vi "Dashboard Main.vi"() -> ()   [LabVIEW 2015]
uses:
  PositionSelect.ctl
  DefenseSelect.ctl
  <vilib>/Utility/miscctls.llb/LVRowAndColumnTypeDef.ctl
  <vilib>/event_ctls.llb/eventvkey.ctl
  <vilib>/Rock Robotics/WPI/Dashboard/WPI_DashboardLogging Global.vi
  <vilib>/Rock Robotics/Network Tables/NT Read Numeric Array.vi
  <vilib>/Rock Robotics/Network Tables/NT Read Boolean.vi
  <vilib>/Rock Robotics/Network Tables/NT Write Numeric Array.vi
  <vilib>/Utility/config.llb/Write Key (String).vi
  <vilib>/Utility/config.llb/Write Key (I32).vi
  <vilib>/Utility/config.llb/NI_LVConfig.lvlib
panel:
  in  "TCP":refnum<k5>
  in  "Rec Mode":enum32{"Stop", "Record", "Playback"}(radio)
  in  "Vision":u16(ring) items=["Camera Off", "USB Camera SW", "USB Camera HW", "IP Camera"]
  out "Camera IP":string
  out "Image Message":string="Timeout in Camera Communications"
  in  "Dashboard Tab":T1(tab)
  in  "Select Auto":string(combo)
  out "NT Connection":bool
  in  "Camera Settings":T2={"Frame Rate"=30, "Compression"=30, "Size"=1} {"Frame Rate" scale=1.0..30.0; "Size" items=["640x480", "320x240", "160x120"]}
  out "MotorChart R":cluster{"Numeric":dbl, "Numeric":dbl}(graph)
  out "MotorChart L":T3(graph)
  out "MotorSliders R":cluster{"MotorSlide1":dbl, "MotorSlide2":dbl} {"MotorSlide2" scale=-1.0..1.0 scale format="%#_2e"; "MotorSlide1" scale=-1.0..1.0 scale format="%#_2e"}
  out "MotorSliders L":T4 {"MotorSlide4 2" scale=0.0..14.0 scale format="%#_2e"; "MotorSlide2" scale=-1.0..1.0 scale format="%#_2e"; "MotorSlide1" scale=-1.0..1.0 scale format="%#_2e"}
  out "JS1 Z":dbl(slide) scale=-1.0..1.0 scale format="%#_2e"
  out "JS1 Graph":cluster{"X":dbl, "Y":dbl}[](graph)
  out "JS1 Buttons":T5
  out "JS2 Z":dbl(slide) scale=-1.0..1.0 scale format="%#_2e"
  out "JS2 Graph":cluster{"X":dbl, "Y":dbl}[](graph)
  out "JS2 Buttons":T5
  out "Mode":T6(ring)=enum."Auto Disabled"
  in  "DB Camera Config":bool
  out "fps":dbl format="%#.1g"
  out "Mbps":dbl format="%#.1g"
  out "Mbps LED":bool
  in  "DB/String 9":string
  in  "DB/String 8":string
  in  "DB/String 7":string
  in  "DB/String 6":string
  in  "DB/String 5":string
  in  "DB/String 4":string
  in  "DB/String 3":string
  in  "DB/String 2":string
  in  "DB/String 1":string
  in  "DB/String 0":string
  in  "DB/Slider 0":dbl(slide) scale=0.0..5.0
  in  "DB/Slider 1":dbl(slide) scale=0.0..5.0
  in  "DB/Slider 2":dbl(slide) scale=0.0..5.0
  in  "DB/Slider 3":dbl(slide) scale=0.0..5.0
  out "DB/LED 3":bool
  out "DB/LED 2":bool
  out "DB/LED 1":bool
  out "DB/LED 0":bool
  in  "DB/Button 3":bool
  in  "DB/Button 2":bool
  in  "DB/Button 1":bool
  in  "DB/Button 0":bool caption="New Name"
  in  "Defense Select":T7
  out "RightEncoder":dbl
  out "LeftEncoder":dbl
  in  "Position Select":T8=enum."1 (Wall)"
  out "Yaw":dbl
  out "Case":dbl
  out "EXIT":bool
  out "CameraSwivel":dbl
  out "CameraTilt":dbl
  out "Defense Select Out":T7
  out "Position Select Out":T8=enum."1 (Wall)"
  out "Roll":dbl
  out "Pitch":dbl
  out "Photoeye\nBeam Broken?":bool
  out "Climb Encoder":dbl
  in  "Test Slider":dbl(slide) scale=0.0..100.0 scale format="%#_3g"
  in  "On/Off":bool caption="Solenoid"
  in  "Test Name":u16(ring) items=["Select the test to run..."]
  in  "Test Tree":string(tree)
  in  "Motor":cluster{"Value":dbl, "Enable":bool} {"Value" scale=-1.0..1.0 scale format="%#_3g"}
  out "Progress":T9 {"Test Progress" scale=0.0..100.0}
  in  "Rev/Fwd":cluster{"Forward":bool, "Reverse":bool}
  in  "Test Ring":u16(ring) items=["Monochrome", "Color"]
  out "Cmd Status":string
  in  "Execute Command":bool
  in  "Command Params":string[][](table)
  in  "Command Selection":i32(listbox)
  in  "CheckList":i32(listbox)
  out "Tree":string(tree)
  out "Camera Image":T10(plugin-control)
  out "Background":bool
  # "Left"
  # "Front"
  # "Right"
  # "Battery"
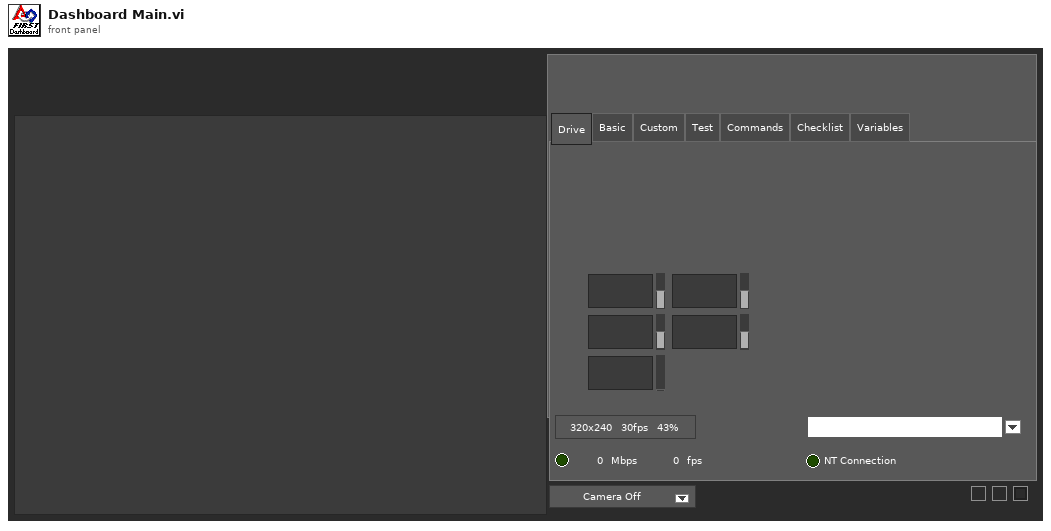
[diagram p1: front panel]
types:
  T1 = enum32{"Drive", "Basic", "Custom", "Test", "Commands", "Checklist", "Variables"}
  T2 = cluster{"Frame Rate":i32, "Compression":i32, "Size":u16}
  T3 = cluster{"Numeric":dbl, "Numeric":dbl, "Battery V":dbl}
  T4 = cluster{"MotorSlide1":dbl, "MotorSlide2":dbl, "MotorSlide4 2":dbl}
  T5 = cluster{bool, bool, bool, bool, bool, bool, bool, bool, bool, bool, bool, bool}
  T6 = enum8{"Tele-Op Disabled", "Tele-Op Enabled", "Auto Disabled", "Auto Enabled", "Test Disabled", "Test Enabled", "Disconnected", "No Code", "E-Stop"}
  T7 = typedef "DefenseSelect.ctl" = enum16{"Low Bar", "Moat", "Rough Terrain", "Rock Wall", "Ramparts", "Portcullis", "Cheval de Frise"}
  T8 = typedef "PositionSelect.ctl" = enum16{"Don't Move", "1 (Wall)", "2", "3", "4", "5", "CrossOnly"}
  T9 = cluster{"Test Progress":u8, "Test Progress Text":string}
  T10 = typedef "IMAQ Image.ctl" = refnum<image>
  T11 = cluster{"IDs":cluster{"RPC field ID":u16, "Unique ID":u16}, "String":string}
  T12 = enum32{"Drive", "Basic", "Custom", "Test", "Checklist", "Variables"}
  T13 = typedef "Image Type" = u32
  T14 = cluster{"Camera Image":refnum<vi>, "Dashboard Tab":refnum<vi>, "Background":refnum<vi>, "Vision":refnum<vi>, "Rec Mode":refnum<vi>, "Test Slider":refnum<vi>, "On/Off ":refnum<vi>, "Test Ring":refnum<vi>, "Rev/Fwd":refnum<vi>, "Test Name":refnum<vi>, "Motor":refnum<vi>, "Progress":refnum<vi>, "CheckList":refnum<vi>, "Tree":refnum<vi>, "Test Tree":refnum<vi>, "Command Params":refnum<vi>, "Command Selection":refnum<vi>, "Execute Command":refnum<vi>, "Cmd Status":refnum<vi>}
  T15 = cluster{"Error Strings":string, "Disable Counts":cluster{u16, u16}, "Rail Faults":cluster{u16, u16, u16}, "Robot IP":string, "DB Mode":u8, "Event Info":cluster{"Name":string, "Type":u8, "Number":u16, "Replay":u8}, "Camera Addr":string}
  T16 = cluster{"Storage":cluster{"Disk Free":u64, "RAM Block":u32, "RAM free":u32}, "CPU Utilization":cluster{"CPU % ISR":sgl, "CPU % Time Crit":sgl, "CPU % Timed Str":sgl, "CPU % High":sgl, "CPU % Above":sgl, "CPU % Normal":sgl, "CPU % Low":sgl}, "CAN":cluster{"% Bus Utilization":sgl, "Bus Off Cnt":u32, "TX_FIFO Full Cnt":u32, "Receive Error Cnt":u8, "Transmit Error Cnt":u8}, "HID":cluster{"HID Outputs":u32, "Rumble Low":u16, "Rumble High":u16}[]}
  T17 = cluster{"Status bits":cluster{"Test Mode":bool, "Autonomous":bool, "Enabled":bool, "Code Start":bool, "Brownout":bool, "Reserved 2":bool, "Reserved 3":bool, "E-Stop":bool}, "Code Trace":cluster{"Disabled":bool, "TeleOp":bool, "Auto":bool, "Test":bool}, "Controller Type":enum16{"unknown", "cRIO", "roboRio"}, "Code?":enum16{"unknown", "noCode", "code"}, "Battery V":dbl}
  T18 = cluster{"Control Bits":cluster{"TestMode":bool, "Autonomous":bool, "Enabled":bool, "FMS Present":bool, bool, bool, bool, "E-Stop":bool}, "Team Station ":u8, "Countdown":sgl, "Joystick Values":cluster{"Axes":dbl[], "Buttons":bool[], "POVs":i16[]}[]}
  T19 = cluster{"Axes":dbl[], "Buttons":bool[], "POVs":i16[]}[]
  T20 = cluster{"Axes":dbl[], "Buttons":bool[], "POVs":i16[]}
  T21 = cluster{"Buttons[0]":bool, "Buttons[1]":bool, "Buttons[2]":bool, "Buttons[3]":bool, "Buttons[4]":bool, "Buttons[5]":bool, "Buttons[6]":bool, "Buttons[7]":bool, "Buttons[8]":bool, "Buttons[9]":bool, "Buttons[10]":bool, "Buttons[11]":bool}
  T22 = typedef "NI_LVConfig.lvlib/Config Data RefNum.ctl" = refnum<k1>
  T23 = cluster{"Operation":enum16{"Update", "Clear"}, "Color Box":u32}[]
  T24 = typedef "eventvkey.ctl" = enum16{"ASCII", "Enter", "Return", "Shift", "Ctrl", "Alt", "Cmd", "Opt", "Caps", "NumLock", "Clear", "Break", "Up", "Down", "Left", "Right", "Insert", "Delete", "Home", "End", "PageUp", "PageDown", "Escape", "Help", "Pause", "ScrollLock", "F1", "F2", "F3", "F4", "F5", "F6", "F7", "F8", "F9", "F10", "F11", "F12", "F13", "F14", "F15", "F16", "F17", "F18", "F19", "F20", "F21", "F22", "F23", "F24", "Play", "VolumeUp", "VolumeDown", "Mute", "Two Byte Char"}
  T25 = cluster{"Image Size":bool, "Image Type":bool, "Pixel Value":bool, "ROI Information":bool, "Zoom Factor":bool}
  T26 = enum8{"Enabled", "Disabled", "Disabled and Grayed Out"}
  T27 = cluster{"Operation":enum16{"Update", "Clear"}, "Color Box":u32}
  T28 = typedef "LVRowAndColumnTypeDef.ctl" = cluster{"Row":i32, "Column":i32}
  T29 = cluster{"Shift":bool, "Ctrl":bool, "Alt":bool, "Cmd":bool, "Opt":bool}
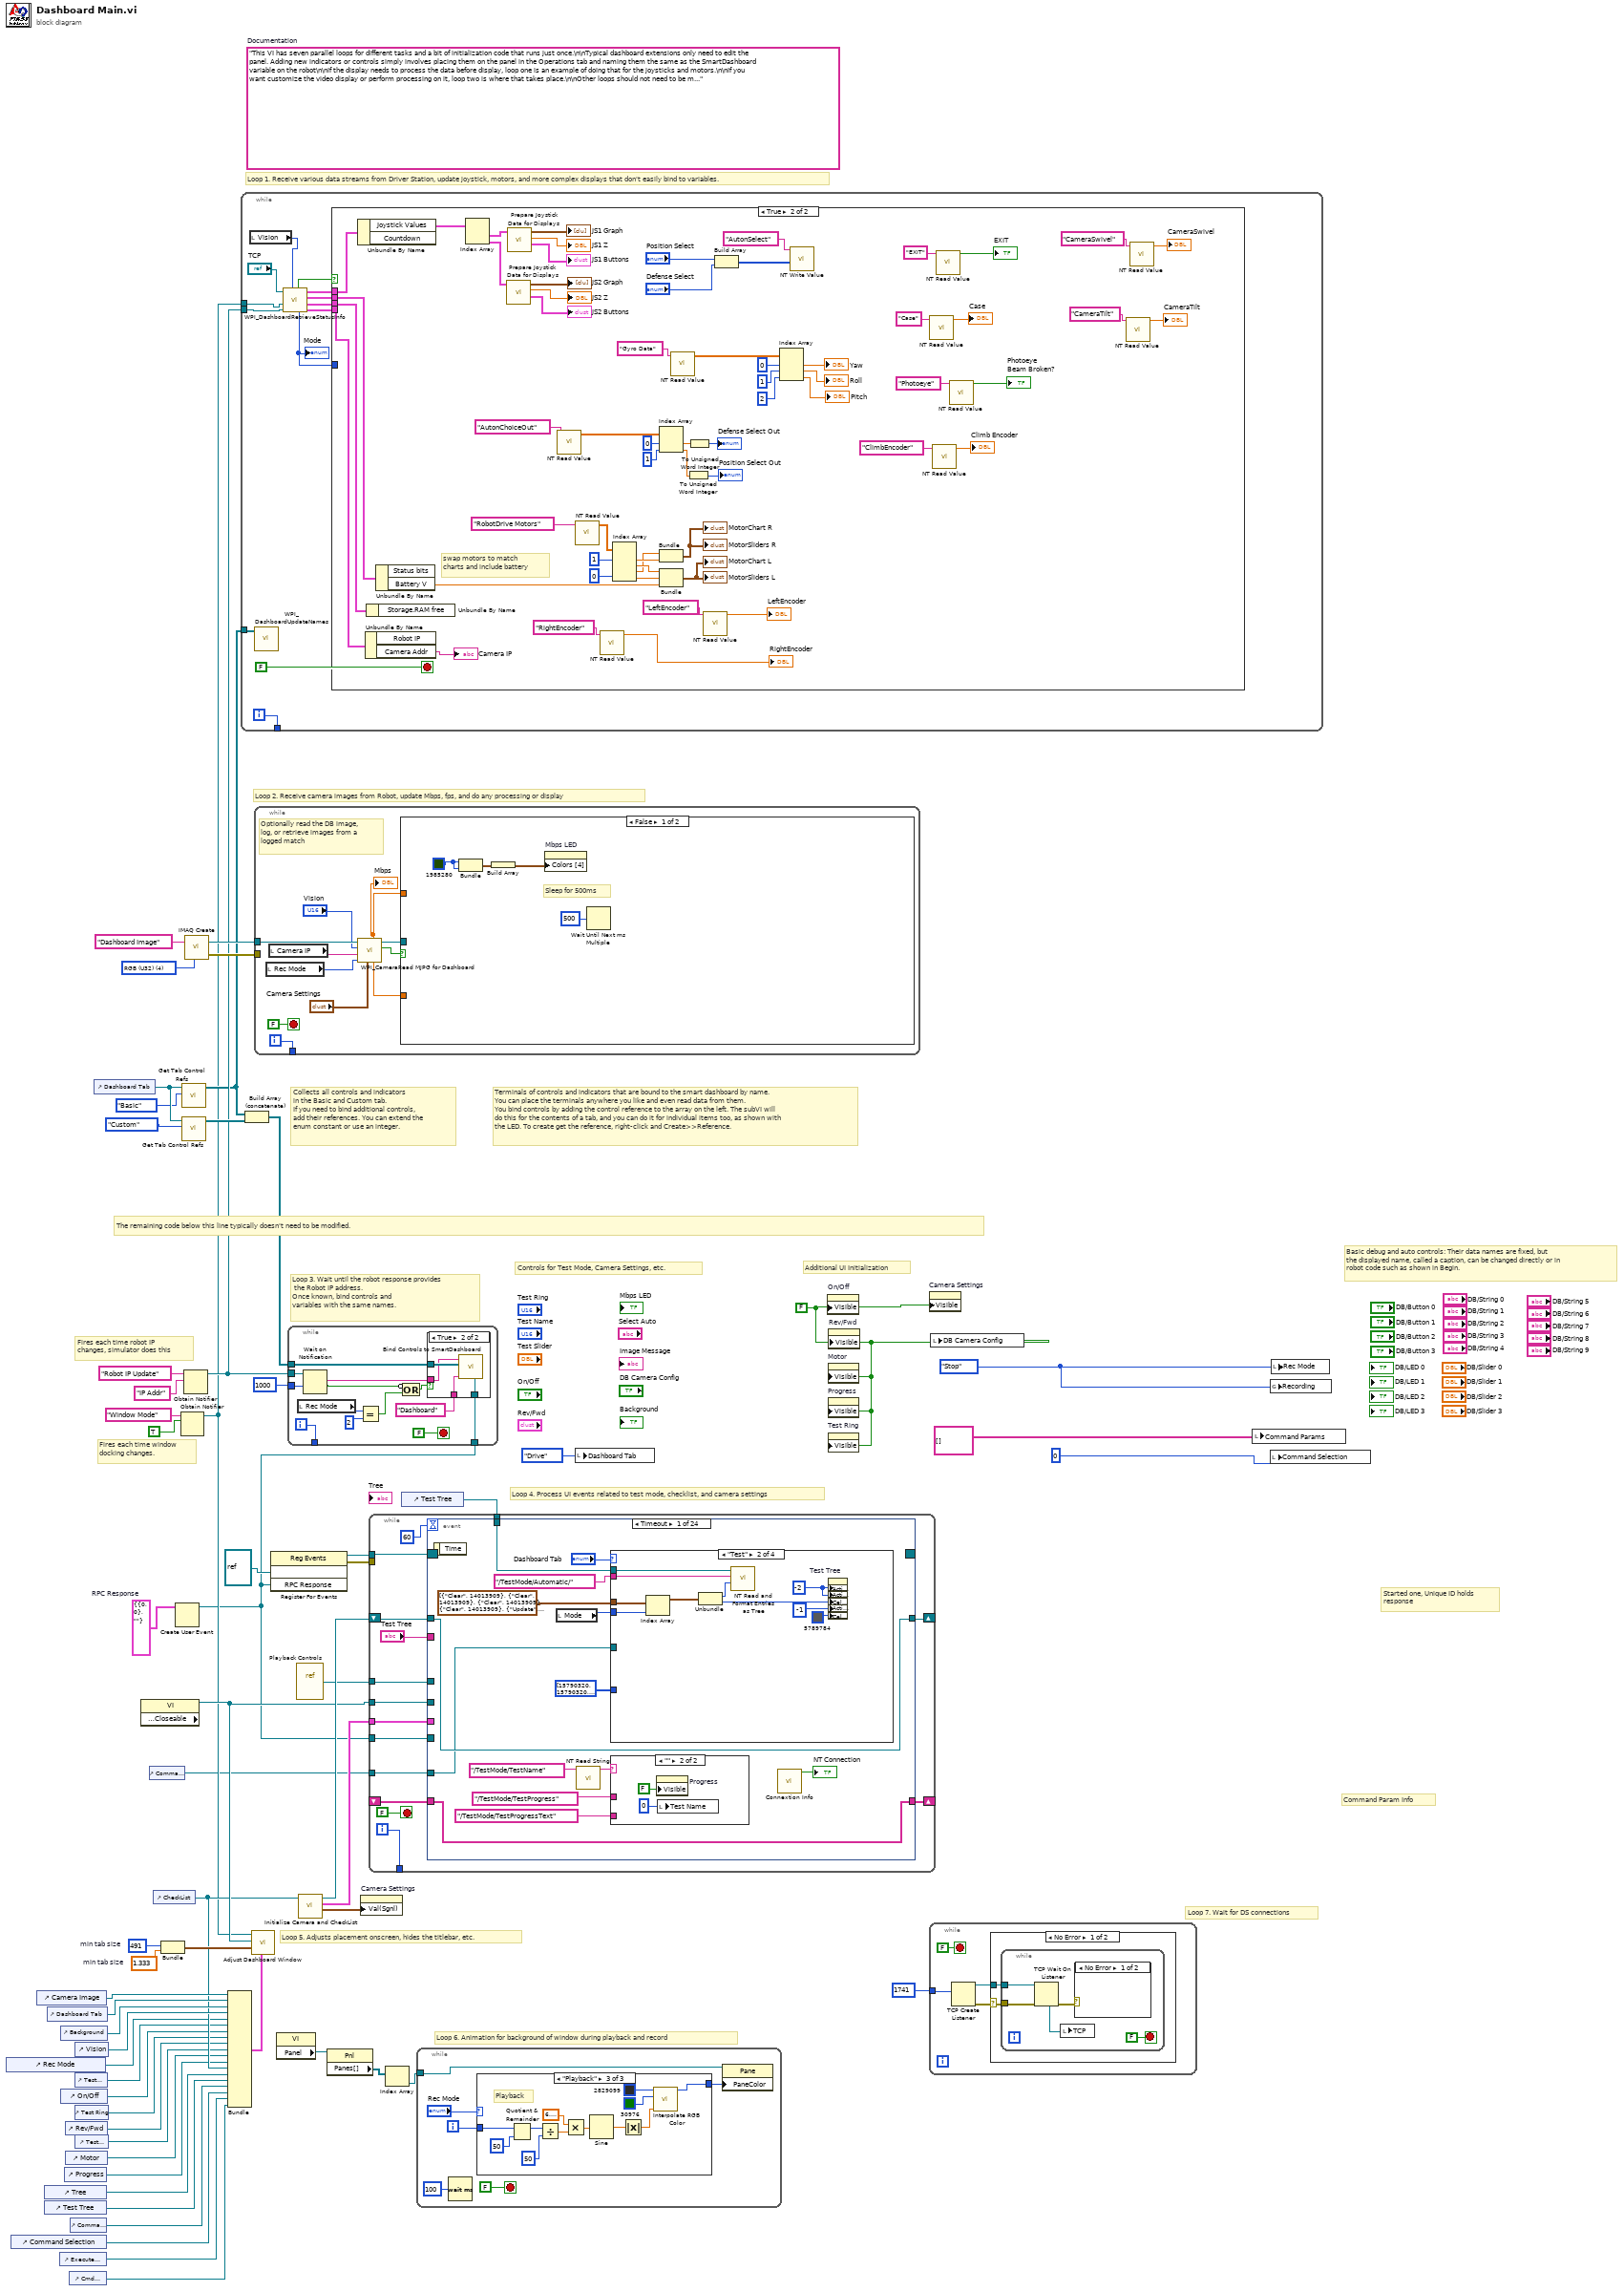
[diagram p0: block diagram]
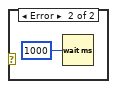
[diagram p2: hidden frame]
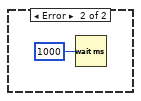
[diagram p3: hidden frame]
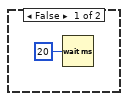
[diagram p4: hidden frame]
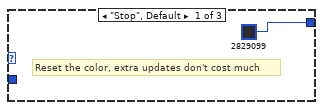
[diagram p5: hidden frame]
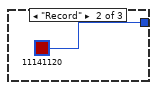
[diagram p6: hidden frame]
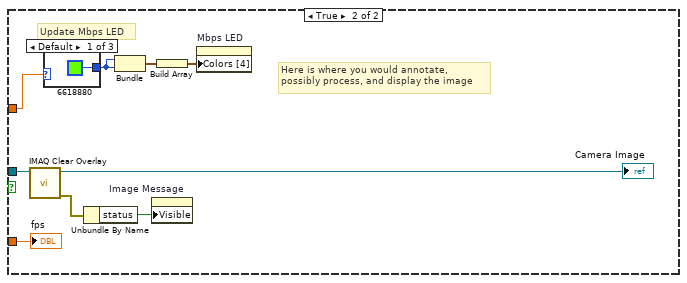
[diagram p8: hidden frame]
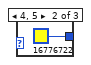
[diagram p9: hidden frame]
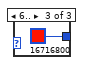
[diagram p10: hidden frame]
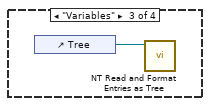
[diagram p12: hidden frame]
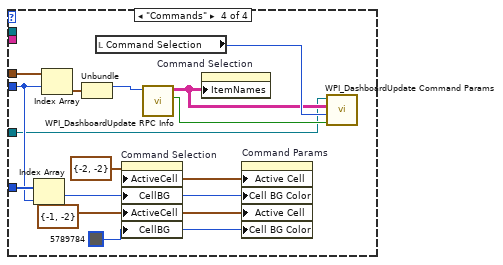
[diagram p13: hidden frame]
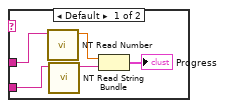
[diagram p14: hidden frame]
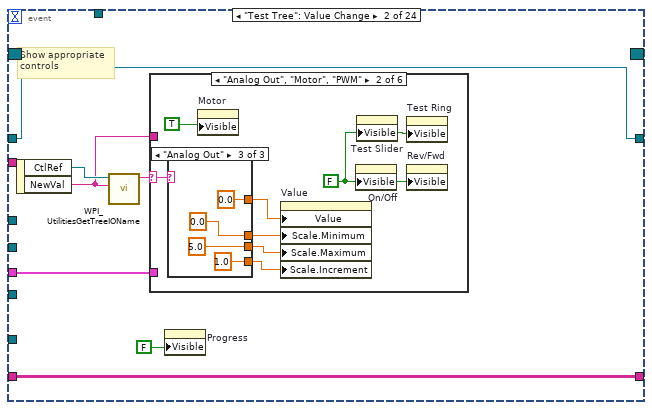
[diagram p15: hidden frame]
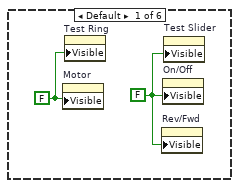
[diagram p16: hidden frame]
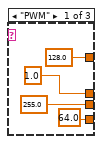
[diagram p17: hidden frame]
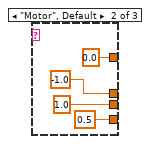
[diagram p18: hidden frame]
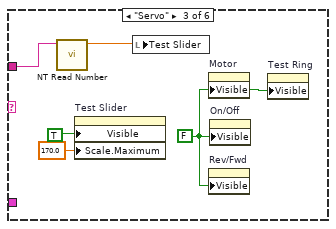
[diagram p19: hidden frame]
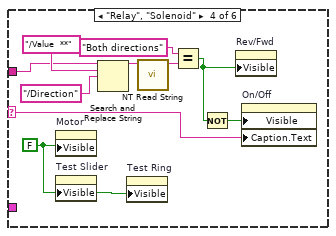
[diagram p20: hidden frame]
diagram:
  w7 = T11 {"IDs"={"RPC field ID"=0, "Unique ID"=0}, "String"=""}  # RPC Response
  w33 = 491  # min tab size
  w32 = 1.333  # min tab size
  w41 = enum32{"Stop", "Record", "Playback"}."Stop" ("Rec Mode")
  w15 = FALSE ("Visible")
  (unwired) "This VI has seven parallel loops for different tasks and a bit of initialization code that runs just once.\n\nTypical dashboard extensions only need to edit the panel. Adding new indicators or controls simply involves placing them on the panel in the Operations tab and naming them the same as the SmartDashboard variable on the robot\n\nIf the display needs to process the data before display, loop one is an example of doing that for the joysticks and motors.\n\nIf you want customize the video display or perform processing on it, loop two is where that takes place.\n\nOther loops should not need to be modified. They are pretty standard, and document the task they perform."  # Documentation
  w61 = T13 4 items=["Grayscale (U8)", "Grayscale (I16)", "Grayscale (SGL)", "Complex (CSG)", "RGB (U32)", "HSL (U32)", "RGB (U64)"] ("Image Type")
  # "Command Param Info"
  # "Started one, Unique ID holds\nresponse"
  # "Loop 7. Wait for DS connections"
  # "Basic debug and auto controls: Their data names are fixed, but\nthe displayed name, called a caption, can be changed directly or in\nrobot code such as shown in Begin."
  # "Controls for Test Mode, Camera Settings, etc."
  # "Additional UI Initialization"
  # "Loop 6. Animation for background of window during playback and record"
  # "Fires each time robot IP\nchanges, simulator does this"
  # "Fires each time window\ndocking changes."
  # "Collects all controls and indicators\nin the Basic and Custom tab.\nIf you need to bind additional controls,\nadd their references. You can extend the\nenum constant or use an integer."
  # "The remaining code below this line typically doesn't need to be modified."
  # "Loop 4. Process UI events related to test mode, checklist, and camera settings"
  # "Terminals of controls and indicators that are bound to the smart dashboard by name.\nYou can place the terminals anywhere you like and even read data from them.\nYou bind controls by adding the control reference to the array on the left. The subVI will\ndo this for the contents of a tab, and you can do it for individual items too, as shown with\nthe LED. To create get the reference, right-click and Create>>Reference."
  # "Loop 3. Wait until the robot response provides\n the Robot IP address.\nOnce known, bind controls and\nvariables with the same names."
  # "Loop 5. Adjusts placement onscreen, hides the titlebar, etc."
  # "Loop 1. Receive various data streams from Driver Station, update joystick, motors, and more complex displays that don't easily bind to variables."
  # "Loop 2. Receive camera images from Robot, update Mbps, fps, and do any processing or display"
  n1 = control-ref of="Rec Mode"() -> (w21:refnum<vi>)
  n2 = control-ref of="Command Selection"() -> (w6:refnum<vi>)
  n3 = control-ref of="Camera Image"() -> (w36:refnum<vi>)
  n4 = control-ref of="Tree"() -> (w25:refnum<vi>)
  n5 = control-ref of="Test Tree"() -> (w24:refnum<vi>)
  n6 = control-ref of="Dashboard Tab"() -> (w35:refnum<vi>)
  n7 = control-ref of="Execute Command"() -> (w8:refnum<vi>)
  n8 = control-ref of="Background"() -> (w30:refnum<vi>)
  n9 = control-ref of="On/Off"() -> (w19:refnum<vi>)
  n10 = control-ref of="Progress"() -> (w16:refnum<vi>)
  n11 = control-ref of="Rev/Fwd"() -> (w17:refnum<vi>)
  n12 = control-ref of="Motor"() -> (w22:refnum<vi>)
  n13 = control-ref of="Cmd Status"() -> (w2:refnum<vi>)
  n14 = control-ref of="Command Params"() -> (w9:refnum<vi>)
  n15 = control-ref of="Test Slider"() -> (w20:refnum<vi>)
  n16 = control-ref of="Vision"() -> (w34:refnum<vi>)
  n17 = control-ref of="Test Ring"() -> (w18:refnum<vi>)
  n18 = control-ref of="Test Name"() -> (w23:refnum<vi>)
  n19 = control-ref of="Dashboard Tab"() -> (w39:refnum<vi>)
  n20 = property class="VI" props=["Front Panel.Closeable"]() -> (reference out=w40:refnum<vi>)  [unwired: 2 in, 2 out]
  n21 = control-ref of="Command Params"() -> (w1:refnum<vi>)
  n22 = control-ref of="CheckList"() -> (w26:refnum<vi>)
  n23 = Bundle("min tab size"=w33, "min tab size"=w32) -> (w31:cluster{"min tab size":i32, "min tab size":dbl})  [unwired: 1 in]
  n24 = Create User Event(user event datatype=w7) -> (user event=w3:refnum<user-event>)  [unwired: 1 in, 1 out]
  n25 = Obtain Notifier(name (unnamed)="Window Mode", notification data type=TRUE) -> (notifier out=w12:refnum<notifier>)  [unwired: 2 in, 2 out]
  n26 = call <vilib>:"Get Tab Control Refs.vi"("Page Index"=T12."Basic" ("Dashboard Tab"), "TabControl in"=w39) -> ("ControlsOnPage"=w13:refnum<vi>[])  [unwired: 9 in]
  n27 = call <vilib>:"Get Tab Control Refs.vi"("Page Index"=T12."Custom" ("Dashboard Tab"), "TabControl in"=w39) -> ("ControlsOnPage"=w38:refnum<vi>[])  [unwired: 9 in]
  n28 = Obtain Notifier(name (unnamed)="Robot IP Update", notification data type="IP Addr" ("name (unnamed)")) -> (notifier out=w14:refnum<notifier>)  [unwired: 2 in, 2 out]
  n29 = call "IMAQ Create"("Image Name"="Dashboard Image", "Image Type"=w61) -> ("New Image"=w59:T10, "error out"=w58:errorcluster)  [unwired: 2 in, 1 out]
  n30 = Bundle("Camera Image"=w36, "Dashboard Tab"=w35, "Background"=w30, "Vision"=w34, "Rec Mode"=w21, "Test Slider"=w20, "On/Off"=w19, "Test Ring"=w18, "Rev/Fwd"=w17, "Test Name"=w23, "Motor"=w22, "Progress"=w16, "CheckList"=w26, "Tree"=w25, "Test Tree"=w24, "Command Params"=w9, "Command Selection"=w6, "Execute Command"=w8, "Cmd Status"=w2) -> (w27:T14)  [unwired: 1 in]
  n31 = while {
    tunnel: [w73] -> _
    tunnel: w14 -> [w67]
    tunnel: w13 -> [w66]
    tunnel: w12 -> [w62]
    i -> [w73]
    stop <- FALSE stop-if-true
    n32 = local read "Vision"() -> (w64:u16)
    n33 = call <vilib>:"WPI_DashboardUpdateNames.vi"("Controls on Tab"=w66) -> ()  [unwired: 11 in]
    n34 = call <vilib>:"WPI_DashboardRetrieveStatusInfo.vi"("Vision"=w64, "Binding Refnum"=w67, "Window Mode Notifier"=w62, "TCP Cnx"="TCP") -> ("Power and Errors"=w68:T15, "Robot Metrics"=w71:T16, "Status Info"=w72:T17, "Control Info"=w69:T18, "Robot Mode"=w65:T6, "Process?"=w70:bool)  [unwired: 2 in]
    "Mode" <- w65
    n35 = case shown="True" w70 {
      tunnel: w72 -> [_ w136]
      tunnel: w71 -> [_ w135]
      tunnel: w69 -> [_ w134]
      tunnel: w68 -> [_ w133]
      tunnel: w65 -> [_ _]
      frame False {
        n36 = Wait (ms)(milliseconds to wait=u32 20) -> ()  [unwired: 1 out]
      }
      frame True {
        # "swap motors to match\ncharts and include battery"
        n37 = Unbundle By Name(w134) -> ("Joystick Values"=w123:T19)  [unwired: 1 out]
        n38 = Unbundle By Name(w133) -> ("Camera Addr"=→"Camera IP":string)  [unwired: 1 out]
        n39 = Unbundle By Name(w135) -> ()  [unwired: 1 out]
        n40 = Unbundle By Name(w136) -> ("Battery V"=w124:dbl)  [unwired: 1 out]
        n41 = Index Array(array=w123) -> (element #1=w122:T20, element #2=w117:T20)  [unwired: 2 in]
        n42 = call "Prepare Joystick Data for Displays.vi"("Joystick Values"=w117) -> ("Buttons"=→"JS2 Buttons":T21, "Z Axis"=→"JS2 Z":dbl, "Cartesian Data"=→"JS2 Graph":cluster{"X axis":dbl, "X axis":dbl}[])  [unwired: 8 in]
        n43 = call "Prepare Joystick Data for Displays.vi"("Joystick Values"=w122) -> ("Buttons"=→"JS1 Buttons":T21, "Z Axis"=→"JS1 Z":dbl, "Cartesian Data"=→"JS1 Graph":cluster{"X axis":dbl, "X axis":dbl}[])  [unwired: 8 in]
        n44 = call-poly <vilib>:"NT Read Value.vi"("Name"="AutonChoiceOut") -> ("Numeric Array"=w91:dbl[])  [unwired: 9 in, 1 out]
        n45 = call-poly <vilib>:"NT Read Value.vi"("Name"="RobotDrive Motors") -> ("Numeric Array"=w112:dbl[])  [unwired: 9 in, 1 out]
        n46 = call-poly <vilib>:"NT Read Value.vi"("Name"="RightEncoder") -> ("Numeric"=→"RightEncoder":dbl)  [unwired: 9 in, 1 out]
        n47 = Index Array(array=w112, index #1=1, index #4=0) -> (element #1=w128:dbl, element #2=w129:dbl, element #3=w127:dbl, element #4=w132:dbl)  [unwired: 2 in]
        n48 = Index Array(array=w91, index #1=0 ("index"), index #2=1 ("index")) -> (element #1=w87:dbl, element #2=w85:dbl)
        n49 = Bundle("Numeric"=w127, "Numeric"=w128) -> (→"MotorChart R" →"MotorSliders R":cluster{"Numeric":dbl, "Numeric":dbl})  [unwired: 1 in]
        n50 = Bundle("Numeric"=w129, "Numeric"=w132, "Battery V"=w124) -> (→"MotorChart L" →"MotorSliders L":T3)  [unwired: 1 in]
        n51 = call-poly <vilib>:"NT Read Value.vi"("Name"="Gyro Data") -> ("Numeric Array"=w110:dbl[])  [unwired: 9 in, 1 out]
        n52 = To Unsigned Word Integer(number=w85) -> (unsigned 16bit integer=→"Position Select Out":u16)
        n53 = To Unsigned Word Integer(number=w87) -> (unsigned 16bit integer=→"Defense Select Out":u16)
        n54 = call-poly <vilib>:"NT Read Value.vi"("Name"="LeftEncoder") -> ("Numeric"=→"LeftEncoder":dbl)  [unwired: 9 in, 1 out]
        n55 = Build Array("Position Select", "Defense Select") -> (w92:u16[])
        n56 = Index Array(array=w110, index #1=0 ("index"), index #2=1 ("index"), index #3=2 ("index")) -> (element #1=→"Yaw":dbl, element #2=→"Roll":dbl, element #3=→"Pitch":dbl)
        n57 = call-poly <vilib>:"NT Write Value.vi"("Numeric Array"=w92, "Name"="AutonSelect") -> ()  [unwired: 9 in, 1 out]
        n58 = call-poly <vilib>:"NT Read Value.vi"("Name"="Case") -> ("Numeric"=→"Case":dbl)  [unwired: 9 in, 1 out]
        n59 = call-poly <vilib>:"NT Read Value.vi"("Name"="ClimbEncoder") -> ("Numeric"=→"Climb Encoder":dbl)  [unwired: 9 in, 1 out]
        n60 = call-poly <vilib>:"NT Read Value.vi"("Name"="EXIT") -> ("Boolean"=→"EXIT":bool)  [unwired: 9 in, 1 out]
        n61 = call-poly <vilib>:"NT Read Value.vi"("Name"="Photoeye") -> ("Boolean"=→"Photoeye\nBeam Broken?":bool)  [unwired: 9 in, 1 out]
        n62 = call-poly <vilib>:"NT Read Value.vi"("Name"="CameraTilt") -> ("Numeric"=→"CameraTilt":dbl)  [unwired: 9 in, 1 out]
        n63 = call-poly <vilib>:"NT Read Value.vi"("Name"="CameraSwivel") -> ("Numeric"=→"CameraSwivel":dbl)  [unwired: 9 in, 1 out]
      }
    }
  }
  n64 = Build Array (concatenate)(w13, w38) -> (w37:refnum<vi>[])
  n65 = call "Adjust Dashboard Window.vi"("Sizing Refnums"=w27, "Size Constraints"=w31, "VI"=w40, "WIn Mode"=w12) -> ()  [unwired: 8 in]
  n66 = while {
    tunnel: w59 -> [w145]
    tunnel: w58 -> [_]
    tunnel: [w146] -> _
    i -> [w146]
    stop <- FALSE stop-if-true
    # "Optionally read the DB image,\nlog, or retrieve images from a\nlogged match"
    n67 = local read "Rec Mode"() -> (w140:enum32{"Stop", "Record", "Playback"})
    n68 = local read "Camera IP"() -> (w138:string)
    n69 = call <vilib>:"WPI_CameraRead MJPG for Dashboard.vi"("Camera Settings"="Camera Settings", "Rec Mode"=w140, "Camera IP"=w138, "Camera Mode"="Vision", "Refnum in"=w145) -> ("Active"=w143:bool, "Refnum out"=w144:T10, "FPS"=w142:dbl, "Bandwidth (Mbps)"=w137:dbl)  [unwired: 3 in]
    "Mbps" <- w137
    n70 = case shown="False" w143 {
      tunnel: w144 -> [_ w155]
      tunnel: w137 -> [_ w154]
      tunnel: w142 -> [_ w152]
      frame False {
        w148 = u32 1985280 ("Color Box")
        # "Sleep for 500ms"
        n71 = Bundle("Color Box"=w148, "Color Box"=w148) -> (w150:cluster{"Color Box":u32, "Color Box":u32})  [unwired: 1 out]
        n72 = Build Array(w150) -> (w149:cluster{"Color Box":u32, "Color Box":u32}[])
        n73 = property on="Mbps LED" class="Bool (strict)"("Colors [4]"=w149) -> ()  [unwired: 2 in, 2 out]
        n74 = Wait Until Next ms Multiple(millisecond multiple=u32 500) -> ()  [unwired: 1 out]
      }
      frame True {
        # "Here is where you would annotate,\npossibly process, and display the image"
        # "Update Mbps LED"
        n75 = call "IMAQ Clear Overlay"("Image"=w155) -> ("error out"=w159:errorcluster, "Image Out"=→"Camera Image":T10)  [unwired: 2 in, 7 out]
        n76 = case shown="Default" w154 {
          tunnel: [u32 6618880 ("Color Box") u32 16776722 ("Color Box") u32 16716800 ("Color Box")] -> w156
          frame Default {
          }
          frame 4, 5 {
          }
          frame 6.. {
          }
        }
        n77 = Unbundle By Name(w159) -> ("status"=w160:bool)
        n78 = Bundle("Color Box"=w156, "Color Box"=w156) -> (w158:cluster{"Color Box":u32, "Color Box":u32})  [unwired: 1 out]
        n79 = property on="Image Message" class="Str"("Visible"=w160) -> ()  [unwired: 2 in, 2 out]
        n80 = Build Array(w158) -> (w157:cluster{"Color Box":u32, "Color Box":u32}[])
        n81 = property on="Mbps LED" class="Bool (strict)"("Colors [4]"=w157) -> ()  [unwired: 2 in, 2 out]
        "fps" <- w152
      }
    }
  }
  n82 = register-events(refnum<vi> refnum, w3) -> (reference out=w45:refnum<event-registration>, error out=w44:errorcluster)  [unwired: 2 in]
  n83 = property class="VI"() -> ("Panel"=w48:refnum<vi>)  [unwired: 2 in, 2 out]
  n84 = while {
    tunnel: w37 -> [w176]
    tunnel: w14 -> [w174]
    tunnel: [w172] -> _
    tunnel: u32 1000 ("milliseconds to wait") -> [w171]
    tunnel: w3 -> [w164]
    i -> [w172]
    stop <- FALSE stop-if-true
    n85 = local read "Rec Mode"() -> (w167:enum32{"Stop", "Record", "Playback"})
    n86 = Wait on Notification(notifier=w174, timeout in ms (-1)=w171) -> (notification=w173:string, timed out?=w169:bool)  [unwired: 2 in, 2 out]
    n87 = Equal?(x=w167, y=u16 2 ("Rec Mode")) -> (x = y?=w168:bool)
    n88 = Compound Arithmetic op=OR(invert w169, w168) -> (w170:bool)
    n89 = case shown="True" w170 {
      tunnel: w176 -> [_ w180]
      tunnel: w173 -> [_ w179]
      tunnel: "Dashboard" -> [_ w178]
      tunnel: w164 -> [_ w177]
      frame False {
      }
      frame True {
        n90 = call <vilib>:"Bind Controls to SmartDashboard.vi"("RPC ref"=w177, "Client Name"=w178, "Bound Control Refs"=w180, "Server IP Address"=w179) -> ()  [unwired: 8 in]
      }
    }
  }
  n91 = vi-ref "Playback Controls.vi"() -> (w46:refnum<vi>)
  n92 = call "Initialize Camera and CheckList.vi"("ListBox in"=w26) -> ("Cluster"=w52:cluster{"value":i32, "value":i32, "index":i32}, "Array"=w53:cluster{string[]}[], "File Refnum"=w51:T22)  [unwired: 8 in]
  n93 = property class="Pnl"(reference=w48) -> ("Panes[]"=w49:refnum<vi>[])  [unwired: 1 in, 2 out]
  n94 = property on="Camera Settings" class="Clust (strict)"("Val(Sgnl)"=w52) -> ()  [unwired: 2 in, 2 out]
  n95 = Index Array(array=w49) -> (element=w47:refnum<vi>)  [unwired: 1 in]
  n96 = control-ref of="Test Tree"() -> (w50:refnum<vi>)
  n97 = while {
    tunnel: w53 -> [w192]
    shift-right: [w191] -> _
    shift-left: w51 -> [w190]
    tunnel: [w189] -> _
    tunnel: w50 -> [w188]
    tunnel: w46 -> [w187]
    tunnel: w45 -> [w186]
    tunnel: w44 -> [_]
    tunnel: w40 -> [w185]
    tunnel: w3 -> [w184]
    tunnel: w1 -> [w183]
    shift-right: [w182] -> _
    shift-left: _ -> [w181]
    i -> [w189]
    stop <- FALSE stop-if-true
    n98 = event shown="[0] Timeout" {
      selector: w186 -> [_ _ _ _ _ _ _ _ _ _ _ _ _ _ _ _ _ _ _ _ _ _ _ _]
      dyn-events: [_ _ _ _ _ _ _ _ _ _ _ _ _ _ _ _ _ _ w501 _ _ _ _ _] -> _
      timeout: u32 60 ("milliseconds to wait") -> [_ _ _ _ _ _ _ _ _ _ _ _ _ _ _ _ _ _ _ _ _ _ _ _]
      tunnel: w188 -> [w205 _ _ _ _ _ _ _ _ _ _ _ _ _ _ _ _ _ _ _ _ _ _ _]
      tunnel: "Test Tree" -> [_ _ _ _ _ _ _ _ _ _ _ _ _ w464 w473 w476 w481 w490 _ _ _ _ _ _]
      tunnel: w192 -> [_ w243 _ _ _ _ _ _ _ _ _ w426 w457 _ _ _ _ _ _ _ _ _ _ _]
      tunnel: [w202 w242 w346 w352 w362 w366 w372 w384 w392 w398 w411 w425 w450 w463 w471 w475 w480 w489 w503 w519 w521 w529 w540 w545] -> w191
      tunnel: w190 -> [w202 w242 w346 w352 w362 w366 w372 w384 w392 w398 w411 w424 w450 w463 w471 w475 w480 w489 w503 w519 w521 w529 w540 w545]
      tunnel: w187 -> [_ _ _ _ _ _ _ _ _ _ _ _ _ _ _ _ _ _ w504 _ w524 _ _ _]
      tunnel: w185 -> [_ _ _ _ _ _ _ _ _ _ _ _ _ _ _ _ _ _ w499 _ _ _ _ _]
      tunnel: w184 -> [_ _ _ _ _ _ _ _ _ _ _ _ _ _ _ _ _ _ w495 _ _ _ _ _]
      tunnel: w183 -> [w197 _ _ _ _ _ w370 _ _ _ _ _ _ _ _ _ _ _ _ _ _ _ _ _]
      tunnel: [w196 w241 w345 w351 w361 w367 w368 w378 w389 w397 w410 w423 w449 w462 w470 w474 w479 w488 w494 w517 w520 w525 w533 w546] -> w182
      tunnel: w181 -> [w196 w241 w345 w351 w361 w367 w368 _ _ w397 w410 w423 w449 w462 w470 w474 w479 w488 w494 w517 w520 w525 w533 w546]
      event Timeout {
        n99 = event-data() -> ()  [unwired: 1 in, 1 out]
        n100 = local read "Mode"() -> (w199:T6)
        n101 = call <vilib>:"NT Read String.vi"("Name"="/TestMode/TestName") -> ("String"=w208:string)  [unwired: 9 in, 1 out]
        n102 = case shown="\"Test\"" "Dashboard Tab" {
          tunnel: w205 -> [_ w219 _ _]
          tunnel: "/TestMode/Automatic/" ("Name Pattern") -> [_ w218 _ _]
          tunnel: T23 [{"Operation"=enum."Clear", "Color Box"=14013909}, {"Operation"=enum."Clear", "Color Box"=14013909}, {"Operation"=enum."Clear", "Color Box"=14013909}, {"Operation"=enum."Clear", "Color Box"=14013909}, {"Operation"=enum."Update", "Color Box"=14013909}, {"Operation"=enum."Update", "Color Box"=16777215}, {"Operation"=enum."Clear", "Color Box"=14013909}, {"Operation"=enum."Clear", "Color Box"=14013909}, {"Operation"=enum."Clear", "Color Box"=14013909}] -> [_ w211 _ w228]
          tunnel: w199 -> [_ w210 _ w227]
          tunnel: u32[] [15790320, 15790320, 15790320, 15790320, 16777215, 16777215, 15790320, 15790320, 15790320] -> [_ _ _ w233]
          tunnel: w197 -> [_ _ _ w221]
          frame "Custom", Default {
          }
          frame "Test" {
            w217 = -2 ("Active Item:Row Number")
            n103 = Index Array(array=w211, index=w210) -> (element=w212:T27)
            n104 = Unbundle(w212) -> ("Operation"=w213:enum16{"Update", "Clear"}, "Color Box"=w214:u32)
            n105 = call <vilib>:"NT Read and Format Entries as Tree.vi"("Operation"=w213, "Name Pattern"=w218, "Tree Refnum"=w219) -> ()  [unwired: 7 in, 2 out]
            n106 = property on="Test Tree" class="Tree (strict)"("Active Item Row Number"=w217, "ActiveColNum"=w217, "CellBG"=w214, "Active Item Row Number"=-1 ("Active Item:Row Number"), "CellBG"=u32 5789784 ("Color Box")) -> ()  [unwired: 2 in, 2 out]
          }
          frame "Variables" {
            n107 = control-ref of="Tree"() -> (w220:refnum<vi>)
            n108 = call <vilib>:"NT Read and Format Entries as Tree.vi"("Tree Refnum"=w220) -> ()  [unwired: 9 in, 2 out]
          }
          frame "Commands" {
            w229 = u32 5789784 ("Color Box")
            w230 = T28 {"Row"=-1, "Column"=-2} ("Active Cell:Active Cell")
            w232 = T28 {"Row"=-2, "Column"=-2} ("Active Cell:Active Cell")
            n109 = Index Array(array=w233, index=w227) -> (element=w231:u32)
            n110 = Index Array(array=w228, index=w227) -> (element=w226:T27)
            n111 = Unbundle(w226) -> ("Operation"=w225:enum16{"Update", "Clear"})  [unwired: 1 out]
            n112 = local read "Command Selection"() -> (w224:i32)
            n113 = property on="Command Selection" class="MCListbox (strict)"("ActiveCell"=w232, "CellBG"=w231, "ActiveCell"=w230, "CellBG"=w229) -> ()  [unwired: 2 in, 2 out]
            n114 = call <vilib>:"WPI_DashboardUpdate RPC Info.vi"("Operation"=w225) -> ("update"=w223:bool, "commands"=w222:string[][])  [unwired: 9 in]
            n115 = property on="Command Selection" class="MCListbox (strict)"("ItemNames"=w222) -> ()  [unwired: 2 in, 2 out]
            n116 = property on="Command Params" class="Tbl (strict)"("Active Cell"=w232, "Cell BG Color"=w231, "Active Cell"=w230, "Cell BG Color"=w229) -> ()  [unwired: 2 in, 2 out]
            n117 = call <vilib>:"WPI_DashboardUpdate Command Params.vi"("Update"=w223, "NewVal"=w224, "Commands"=w222, "Param Tbl"=w221) -> ()  [unwired: 7 in, 1 out]
          }
        }
        n118 = case shown="\"\"" w208 {
          tunnel: "/TestMode/TestProgress" ("Name") -> [w235 _]
          tunnel: "/TestMode/TestProgressText" ("Name") -> [w234 _]
          frame Default {
            n119 = call <vilib>:"NT Read Number.vi"("Name"=w235) -> ("Numeric"=w236:dbl)  [unwired: 9 in, 1 out]
            n120 = call <vilib>:"NT Read String.vi"("Name"=w234) -> ("String"=w237:string)  [unwired: 9 in, 1 out]
            n121 = Bundle("Numeric"=w236, "String"=w237) -> (→"Progress":cluster{"Numeric":dbl, "String":string})  [unwired: 1 in]
          }
          frame "" {
            n122 = property on="Progress" class="Clust (strict)"("Visible"=FALSE) -> ()  [unwired: 2 in, 2 out]
            n123 = local write "Test Name"(u16 0) -> ()
          }
        }
        n124 = call <vilib>:"Connextion Info.vi"() -> ("Connected"=→"NT Connection":bool)  [unwired: 10 in, 1 out]
      }
      event "Test Tree": Value Change {
        # "Show appropriate\ncontrols"
        n125 = event-data() -> ("CtlRef"=w246:refnum<vi>, "NewVal"=w244:string)  [unwired: 1 in]
        n126 = call <vilib>:"WPI_UtilitiesGetTreeIOName.vi"("NewVal"=w244, "TreeControl in"=w246) -> ("I/O Name"=w247:string)  [unwired: 9 in]
        n127 = case shown="\"Analog Out\", \"Motor\", \"PWM\"" w247 {
          selector: w247 -> [_ w254 _ w276 w285 _]
          tunnel: w244 -> [_ _ w273 w275 _ w292]
          tunnel: w243 -> [_ _ _ _ _ w291]
          frame Default {
            w249 = FALSE ("Visible")
            w248 = FALSE ("Visible")
            n128 = property on="Motor" class="Clust (strict)"("Visible"=w248) -> ()  [unwired: 2 in, 2 out]
            n129 = property on="Test Ring" class="Ring (strict)"("Visible"=w248) -> ()  [unwired: 2 in, 2 out]
            n130 = property on="Rev/Fwd" class="Clust (strict)"("Visible"=w249) -> ()  [unwired: 2 in, 2 out]
            n131 = property on="On/Off" class="Bool (strict)"("Visible"=w249) -> ()  [unwired: 2 in, 2 out]
            n132 = property on="Test Slider" class="Slide (strict)"("Visible"=w249) -> ()  [unwired: 2 in, 2 out]
          }
          frame "Analog Out", "Motor", "PWM" {
            w255 = FALSE ("Visible")
            n133 = case shown="\"Analog Out\"" w254 {
              tunnel: [1.0 ("Value") -1.0 ("Value") 0.0 ("Value")] -> w253
              tunnel: [255.0 ("Value") 1.0 ("Value") 5.0 ("Value")] -> w252
              tunnel: [128.0 ("Value") 0.0 ("Value") 0.0 ("Value")] -> w251
              tunnel: [64.0 ("Value") 0.5 ("Value") 1.0 ("Value")] -> w250
              frame "PWM" {
              }
              frame "Motor", Default {
              }
              frame "Analog Out" {
              }
            }
            n134 = property on="Motor" class="Clust (strict)"("Visible"=TRUE) -> ()  [unwired: 2 in, 2 out]
            n135 = property on="Value" class="Slide (strict)"("Value"=w251, "Scale.Minimum"=w253, "Scale.Maximum"=w252, "Scale.Increment"=w250) -> ()  [unwired: 2 in, 2 out]
            n136 = property on="On/Off" class="Bool (strict)"("Visible"=w255) -> ()  [unwired: 2 in, 2 out]
            n137 = property on="Test Slider" class="Slide (strict)"("Visible"=w255) -> ()  [unwired: 2 in, 2 out]
            n138 = property on="Test Ring" class="Ring (strict)"("Visible"=w255) -> ()  [unwired: 2 in, 2 out]
            n139 = property on="Rev/Fwd" class="Clust (strict)"("Visible"=w255) -> ()  [unwired: 2 in, 2 out]
          }
          frame "Servo" {
            w271 = FALSE ("Visible")
            n140 = call <vilib>:"NT Read Number.vi"("Name"=w273) -> ("Numeric"=w272:dbl)  [unwired: 9 in, 1 out]
            n141 = property on="Test Slider" class="Slide (strict)"("Visible"=TRUE, "Scale.Maximum"=170.0 ("Scale.Range:Maximum")) -> ()  [unwired: 2 in, 2 out]
            n142 = local write "Test Slider"(w272) -> ()
            n143 = property on="Motor" class="Clust (strict)"("Visible"=w271) -> ()  [unwired: 2 in, 2 out]
            n144 = property on="Rev/Fwd" class="Clust (strict)"("Visible"=w271) -> ()  [unwired: 2 in, 2 out]
            n145 = property on="On/Off" class="Bool (strict)"("Visible"=w271) -> ()  [unwired: 2 in, 2 out]
            n146 = property on="Test Ring" class="Ring (strict)"("Visible"=w271) -> ()  [unwired: 2 in, 2 out]
          }
          frame "Relay", "Solenoid" {
            w274 = FALSE ("Visible")
            n147 = property on="Motor" class="Clust (strict)"("Visible"=w274) -> ()  [unwired: 2 in, 2 out]
            n148 = property on="Test Slider" class="Slide (strict)"("Visible"=w274) -> ()  [unwired: 2 in, 2 out]
            n149 = Search and Replace String(input string=w275, search string="/Value  **", replace string="/Direction") -> (result string=w281:string)  [unwired: 5 in, 3 out]
            n150 = property on="Test Ring" class="Ring (strict)"("Visible"=w274) -> ()  [unwired: 2 in, 2 out]
            n151 = call <vilib>:"NT Read String.vi"("Name"=w281) -> ("String"=w279:string)  [unwired: 9 in, 1 out]
            n152 = Equal?(x="Both directions", y=w279) -> (x = y?=w277:bool)
            n153 = Not(x=w277) -> (.not. x?=w278:bool)
            n154 = property on="Rev/Fwd" class="Clust (strict)"("Visible"=w277) -> ()  [unwired: 2 in, 2 out]
            n155 = property on="On/Off" class="Bool (strict)"("Visible"=w278, "Caption.Text"=w276) -> ()  [unwired: 2 in, 2 out]
          }
          frame "Compressor", "Digital Out" {
            w284 = FALSE ("Visible")
            # "Get direction and finish"
            n156 = property on="Motor" class="Clust (strict)"("Visible"=w284) -> ()  [unwired: 2 in, 2 out]
            n157 = property on="Test Slider" class="Slide (strict)"("Visible"=w284) -> ()  [unwired: 2 in, 2 out]
            n158 = property on="Test Ring" class="Ring (strict)"("Visible"=w284) -> ()  [unwired: 2 in, 2 out]
            n159 = property on="On/Off" class="Bool (strict)"("Visible"=TRUE, "Caption.Text"=w285) -> ()  [unwired: 2 in, 2 out]
            n160 = property on="Rev/Fwd" class="Clust (strict)"("Visible"=FALSE) -> ()  [unwired: 2 in, 2 out]
          }
          frame "Camera" {
            n161 = call <vilib>:"Get Last Path Segment.vi"("String in"=w292) -> ("String out"=w293:string)  [unwired: 10 in]
            n162 = property on="On/Off" class="Bool (strict)"("Visible"=FALSE) -> ()  [unwired: 2 in, 2 out]
            n163 = property on="Motor" class="Clust (strict)"("Visible"=FALSE) -> ()  [unwired: 2 in, 2 out]
            n164 = property on="Rev/Fwd" class="Clust (strict)"("Visible"=FALSE) -> ()  [unwired: 2 in, 2 out]
            n165 = case shown="\"White Balance  **\"" w293 {
              tunnel: w292 -> [w299 w308 w317 w326 w335 _ w341]
              tunnel: w291 -> [w297 w305 w314 w323 w332 _ _]
              frame "Size  **" {
                n166 = Index Array(array=w297) -> (element=w296:cluster{string[]})  [unwired: 1 in]
                n167 = call <vilib>:"NT Read String.vi"("Name"=w299) -> ("String"=w298:string)  [unwired: 9 in, 1 out]
                n168 = Unbundle(w296) -> (w294:string[])
                n169 = Match First String(2:w294, 3:w298) -> (0:w295:i32)  [unwired: 1 out]
                n170 = property on="Test Ring" class="Ring (strict)"("Value"=w295, "Strings []"=w294) -> ()  [unwired: 2 in, 2 out]
                n171 = property on="Test Ring" class="Ring (strict)"("Visible"=TRUE) -> ()  [unwired: 2 in, 2 out]
                n172 = property on="Test Slider" class="Slide (strict)"("Visible"=FALSE) -> ()  [unwired: 2 in, 2 out]
              }
              frame "White Balance  **" {
                n173 = Index Array(array=w305, index=1) -> (element=w306:cluster{string[]})
                n174 = call <vilib>:"NT Read String.vi"("Name"=w308) -> ("String"=w307:string)  [unwired: 9 in, 1 out]
                n175 = Unbundle(w306) -> (w303:string[])
                n176 = Match First String(2:w303, 3:w307) -> (0:w302:i32)  [unwired: 1 out]
                n177 = property on="Test Ring" class="Ring (strict)"("Value"=w302, "Strings []"=w303) -> ()  [unwired: 2 in, 2 out]
                n178 = property on="Test Ring" class="Ring (strict)"("Visible"=TRUE) -> ()  [unwired: 2 in, 2 out]
                n179 = property on="Test Slider" class="Slide (strict)"("Visible"=FALSE) -> ()  [unwired: 2 in, 2 out]
              }
              frame "Exposure  **" {
                n180 = Index Array(array=w314, index=2) -> (element=w315:cluster{string[]})
                n181 = call <vilib>:"NT Read String.vi"("Name"=w317) -> ("String"=w316:string)  [unwired: 9 in, 1 out]
                n182 = Unbundle(w315) -> (w311:string[])
                n183 = Match First String(2:w311, 3:w316) -> (0:w312:i32)  [unwired: 1 out]
                n184 = property on="Test Ring" class="Ring (strict)"("Value"=w312, "Strings []"=w311) -> ()  [unwired: 2 in, 2 out]
                n185 = property on="Test Ring" class="Ring (strict)"("Visible"=TRUE) -> ()  [unwired: 2 in, 2 out]
                n186 = property on="Test Slider" class="Slide (strict)"("Visible"=FALSE) -> ()  [unwired: 2 in, 2 out]
              }
              frame "Exposure Priority  **" {
                n187 = Index Array(array=w323, index=3) -> (element=w324:cluster{string[]})
                n188 = call <vilib>:"NT Read String.vi"("Name"=w326) -> ("String"=w325:string)  [unwired: 9 in, 1 out]
                n189 = Unbundle(w324) -> (w320:string[])
                n190 = Match First String(2:w320, 3:w325) -> (0:w321:i32)  [unwired: 1 out]
                n191 = property on="Test Ring" class="Ring (strict)"("Value"=w321, "Strings []"=w320) -> ()  [unwired: 2 in, 2 out]
                n192 = property on="Test Ring" class="Ring (strict)"("Visible"=TRUE) -> ()  [unwired: 2 in, 2 out]
                n193 = property on="Test Slider" class="Slide (strict)"("Visible"=FALSE) -> ()  [unwired: 2 in, 2 out]
              }
              frame "Color Enable  **" {
                n194 = Index Array(array=w332, index=4) -> (element=w333:cluster{string[]})
                n195 = call <vilib>:"NT Read String.vi"("Name"=w335) -> ("String"=w334:string)  [unwired: 9 in, 1 out]
                n196 = Unbundle(w333) -> (w329:string[])
                n197 = Match First String(2:w329, 3:w334) -> (0:w330:i32)  [unwired: 1 out]
                n198 = property on="Test Ring" class="Ring (strict)"("Value"=w330, "Strings []"=w329) -> ()  [unwired: 2 in, 2 out]
                n199 = property on="Test Ring" class="Ring (strict)"("Visible"=TRUE) -> ()  [unwired: 2 in, 2 out]
                n200 = property on="Test Slider" class="Slide (strict)"("Visible"=FALSE) -> ()  [unwired: 2 in, 2 out]
              }
              frame Default {
                n201 = property on="Test Ring" class="Ring (strict)"("Visible"=FALSE) -> ()  [unwired: 2 in, 2 out]
                n202 = property on="Test Slider" class="Slide (strict)"("Visible"=FALSE) -> ()  [unwired: 2 in, 2 out]
              }
              frame "Brightness  **", "Color Level  **", "Compression  **", "FPS  **", "Sharpness  **" {
                n203 = call <vilib>:"NT Read Number.vi"("Name"=w341) -> ("Numeric"=w340:dbl)  [unwired: 9 in, 1 out]
                n204 = local write "Test Slider"(w340) -> ()
                n205 = property on="Test Slider" class="Slide (strict)"("Visible"=TRUE, "Scale.Maximum"=100.0 ("Scale.Range:Maximum")) -> ()  [unwired: 2 in, 2 out]
                n206 = property on="Test Ring" class="Ring (strict)"("Visible"=FALSE) -> ()  [unwired: 2 in, 2 out]
              }
            }
          }
        }
        n207 = property on="Progress" class="Clust (strict)"("Visible"=FALSE) -> ()  [unwired: 2 in, 2 out]
      }
      event "Test Name": Mouse Enter {
        # "Populate the ring with the list of tests"
        n208 = event-data() -> ()  [unwired: 1 in, 1 out]
        n209 = call <vilib>:"NT Read String Array.vi"("Name"="/TestMode/TestList") -> ("String Array"=w350:string[])  [unwired: 9 in, 1 out]
        n210 = Build Array (concatenate)("Select the test to run...", w350) -> (w349:string[])
        n211 = property on="Test Name" class="Ring (strict)"("Strings []"=w349) -> ()  [unwired: 2 in, 2 out]
      }
      event "Test Name": Value Change {
        w353 = FALSE ("Visible")
        # "Tell the robot the test name to run"
        n212 = event-data() -> ("NewVal"=w357:u16)  [unwired: 1 in]
        n213 = property on="Test Name" class="Ring (strict)"() -> ("Strings []"=w358:string[])  [unwired: 2 in, 2 out]
        n214 = local write "Progress"(T9 {"Test Progress"=0, "Test Progress Text"=""} ("Progress")) -> ()
        n215 = Index Array(array=w358, index=w357) -> (element=w356:string)
        n216 = call <vilib>:"NT Write String.vi"("String"=w356, "Name"="/TestMode/TestName") -> ()  [unwired: 9 in, 1 out]
        n217 = property on="Progress" class="Clust (strict)"("Visible"=TRUE) -> ()  [unwired: 2 in, 2 out]
        n218 = property on="Motor" class="Clust (strict)"("Visible"=w353) -> ()  [unwired: 2 in, 2 out]
        n219 = property on="Test Slider" class="Slide (strict)"("Visible"=w353) -> ()  [unwired: 2 in, 2 out]
        n220 = property on="On/Off" class="Bool (strict)"("Visible"=w353) -> ()  [unwired: 2 in, 2 out]
        n221 = property on="Rev/Fwd" class="Clust (strict)"("Visible"=w353) -> ()  [unwired: 2 in, 2 out]
        n222 = property on="Test Ring" class="Ring (strict)"("Visible"=w353) -> ()  [unwired: 2 in, 2 out]
      }
      event "Select Auto": Mouse Enter {
        # "Populate the combo box with the list of autonomous options"
        n223 = event-data() -> ()  [unwired: 1 in, 1 out]
        n224 = call <vilib>:"NT Read String Array.vi"("Name"="Auto List") -> ("String Array"=w360:string[])  [unwired: 9 in, 1 out]
        n225 = property on="Select Auto" class="CmbBox"("Strings[]"=w360) -> ()  [unwired: 2 in, 2 out]
      }
      event "Select Auto": Value Change {
        # "User modified the Auto Selection. Write to NT variable so robot knows."
        n226 = event-data() -> ("NewVal"=w364:string)  [unwired: 1 in]
        n227 = call <vilib>:"NT Write String.vi"("String"=w364, "Name"="Auto Selector") -> ()  [unwired: 9 in, 1 out]
      }
      event "Command Selection": Value Change {
        # "Get the params and show in table"
        n228 = event-data() -> ("NewVal"=w371:i32)  [unwired: 1 in]
        n229 = property on="Command Selection" class="MCListbox (strict)"() -> ("ItemNames"=w369:string[][])  [unwired: 2 in, 2 out]
        n230 = call <vilib>:"WPI_DashboardUpdate Command Params.vi"("NewVal"=w371, "Commands"=w369, "Param Tbl"=w370) -> ()  [unwired: 8 in, 1 out]
      }
      event "Execute Command": Value Change {
        # "Started one, Unique ID holds\nresponse"
        n231 = event-data() -> ()  [unwired: 1 in, 1 out]
        n232 = property on="Command Selection" class="MCListbox (strict)"() -> ("ItemNames"=w383:string[][])  [unwired: 2 in, 2 out]
        n233 = Index Array(array=w383, index (row)="Command Selection", index (col)=0) -> (element=w381:string)
        n234 = call <vilib>:"Invoke Commands.vi"("Command Params"="Command Params", "Function Name"=w381) -> ("Params"=w377:u8, "Started"=w376:bool)  [unwired: 7 in, 1 out]
        n235 = Array Subset(array="Command Params", length (row)=w377) -> (w378:string[][])  [unwired: 3 in]
        n236 = Select(t="Executing" ("Cmd Status"), s=w376, f="" ("Cmd Status")) -> (s? t:f=→"Cmd Status":string)
      }
      event "Command Selection": Double Click {
        n237 = event-data() -> ("Row"=w393:i32)  [unwired: 1 in]
        n238 = property on="Command Selection" class="MCListbox (strict)"() -> ("ItemNames"=w396:string[][])  [unwired: 2 in, 2 out]
        n239 = local read "Command Params"() -> (w391:string[][])
        n240 = Index Array(array=w396, index (row)=w393, index (col)=0) -> (element=w394:string)
        n241 = call <vilib>:"Invoke Commands.vi"("Command Params"=w391, "Function Name"=w394) -> ("Params"=w390:u8, "Started"=w385:bool)  [unwired: 7 in, 1 out]
        n242 = Array Subset(array=w391, length (row)=w390) -> (w389:string[][])  [unwired: 3 in]
        n243 = Select(t="Executing" ("Cmd Status"), s=w385, f="" ("Cmd Status")) -> (s? t:f=w386:string)
        n244 = local write "Cmd Status"(w386) -> ()
      }
      event "CheckList": Double Click {
        # "Shift clears all"
        # "Update symbols on the listbox"
        n245 = event-data() -> ("PlatMods.Shift"=w399:bool, "Row"=w401:i32)  [unwired: 1 in]
        n246 = case shown="True" w399 {
          tunnel: w401 -> [w405 _]
          tunnel: 1 -> [w404 _]
          frame False {
            n247 = property on="CheckList" class="LstBox (strict)"() -> ("Item Symbols"=w403:i32[])  [unwired: 2 in, 2 out]
            n248 = Replace Array Subset(array=w403, new element=w404, index=w405) -> (w402:i32[])
            n249 = property on="CheckList" class="LstBox (strict)"("Item Symbols"=w402) -> ()  [unwired: 2 in, 2 out]
          }
          frame True {
            w406 = 0 ("Top Row")
            n250 = property on="CheckList" class="LstBox (strict)"() -> ("Number of Rows"=w408:u32)  [unwired: 2 in, 2 out]
            n251 = Initialize Array(0, w408) -> (w407:i32[])
            n252 = property on="CheckList" class="LstBox (strict)"("Top Row"=w406, "Value"=w406, "Item Symbols"=w407) -> ()  [unwired: 2 in, 2 out]
          }
        }
      }
      event "CheckList": Key Down {
        # "Update symbols on the listbox\nLeft and right keys check and uncheck"
        n253 = event-data() -> ("VKey"=w413:T24)  [unwired: 1 in]
        n254 = case shown="\"Left\", \"Right\"" w413 {
          selector: w413 -> [w418 _]
          tunnel: eventvkey."Left" ("VKey") -> [w416 _]
          frame "Left", "Right" {
            n255 = Equal?(x=w416, y=w418) -> (x = y?=w417:bool)
            n256 = Select(t=0, s=w417, f=1) -> (s? t:f=w419:i32)
            n257 = property on="CheckList" class="LstBox (strict)"() -> ("Item Symbols"=w422:i32[])  [unwired: 2 in, 2 out]
            n258 = Replace Array Subset(array=w422, new element=w419, index="CheckList") -> (w421:i32[])
            n259 = property on="CheckList" class="LstBox (strict)"("Item Symbols"=w421) -> ()  [unwired: 2 in, 2 out]
          }
          frame Default {
          }
        }
      }
      event "DB Camera Config": Value Change {
        # "Show or hide the cluster of controls, store in ini file"
        n260 = event-data() -> ("NewVal"=w427:bool)  [unwired: 1 in]
        n261 = case shown="False" w427 {
          tunnel: w426 -> [w436 _]
          tunnel: [w429 w447] -> w425
          tunnel: w424 -> [w428 w447]
          frame False {
            w443 = "Camera"
            w446 = FALSE ("Visible")
            n262 = local read "Camera Settings"() -> (w435:T2)
            n263 = Index Array(array=w436) -> (element=w439:cluster{string[]})  [unwired: 1 in]
            n264 = Unbundle(w435) -> ("Frame Rate"=w434:i32, "Compression"=w433:i32, "Size"=w437:u16)
            n265 = Unbundle(w439) -> (w438:string[])
            n266 = Index Array(array=w438, index=w437) -> (element=w432:string)
            n267 = call-poly <vilib>:"Write Key.vi"("section"=w443, "value"=w432, "key"="Size", "refnum"=w428) -> ("refnum out"=w445:T22)  [unwired: 2 in, 5 out]
            n268 = call-poly <vilib>:"Write Key.vi"("section"=w443, "value"=w434, "key"="FrameRate", "refnum"=w445) -> ("refnum out"=w444:T22)  [unwired: 1 in, 6 out]
            n269 = property on="Camera Settings" class="Clust (strict)"("Visible"=w446) -> ()  [unwired: 2 in, 2 out]
            n270 = local write "DB Camera Config"(w446) -> ()
            n271 = call-poly <vilib>:"Write Key.vi"("section"=w443, "value"=w433, "key"="Compression", "refnum"=w444) -> ("refnum out"=w430:T22)  [unwired: 1 in, 6 out]
            n272 = call <vilib>:"Close Config Data.vi"("refnum"=w430) -> ("file path"=w431:path)  [unwired: 2 in, 8 out]
            n273 = call <vilib>:"Open Config Data.vi"("configuration file path"=w431) -> ("refnum"=w429:T22)  [unwired: 8 in, 2 out]
          }
          frame True {
            n274 = property on="Camera Settings" class="Clust (strict)"("Visible"=TRUE) -> ()  [unwired: 2 in, 2 out]
          }
        }
      }
      event "Camera Settings": Value Change {
        # "Update summary string when any elements of DB camera change"
        n275 = event-data() -> ("NewVal"=w461:T2)  [unwired: 1 in]
        n276 = Index Array(array=w457) -> (element=w456:cluster{string[]})  [unwired: 1 in]
        n277 = Unbundle(w461) -> ("Frame Rate"=w452:i32, "Compression"=w451:i32, "Size"=w454:u16)
        n278 = Unbundle(w456) -> (w455:string[])
        n279 = Index Array(array=w455, index=w454) -> (element=w453:string)
        n280 = Format Into String(format string="%s   %dfps   %d%%", w453, w452, w451) -> (resulting string=w458:string)  [unwired: 2 in, 1 out]
        n281 = Build Array(w458) -> (w459:string[])
        n282 = property on="DB Camera Config" class="Bool (strict)"("Strings [4]"=w459) -> ()  [unwired: 2 in, 2 out]
      }
      event "Motor.Enable": Value Change {
        # "When the test mode otor enable helper is set, update that\ntree row item's value"
        n283 = event-data() -> ("NewVal"=w468:bool)  [unwired: 1 in]
        n284 = Unbundle("Motor") -> ("Value"=w467:dbl)  [unwired: 1 out]
        n285 = Select(t=w467, s=w468, f=0.0) -> (s? t:f=w465:dbl)
        n286 = call <vilib>:"NT Write Number.vi"("Numeric"=w465, "Name"=w464) -> ()  [unwired: 9 in, 1 out]
      }
      event "Test Slider": Value Change {
        # "When the test mode slider helper is set, update that\ntree row item's value"
        n287 = event-data() -> ("NewVal"=w472:dbl)  [unwired: 1 in]
        n288 = call <vilib>:"NT Write Number.vi"("Numeric"=w472, "Name"=w473) -> ()  [unwired: 9 in, 1 out]
      }
      event "On/Off": Value Change {
        # "When the test mode on/off helper value is set, update that\ntree row item's value"
        n289 = event-data() -> ("NewVal"=w478:bool)  [unwired: 1 in]
        n290 = Boolean To (0,1)(Boolean=w478) -> (0, 1=w477:i16)
        n291 = call <vilib>:"NT Write Number.vi"("Numeric"=w477, "Name"=w476) -> ()  [unwired: 9 in, 1 out]
      }
      event "Rev/Fwd": Value Change {
        # "When the test mode helper value for relays is set, update that\ntree row item's value"
        n292 = event-data() -> ("NewVal.Forward"=w487:bool, "NewVal.Reverse"=w486:bool)  [unwired: 1 in]
        n293 = Boolean To (0,1)(Boolean=w487) -> (0, 1=w483:i16)
        n294 = Boolean To (0,1)(Boolean=w486) -> (0, 1=w485:i16)
        n295 = Negate(x=w485) -> (-x=w484:i16)
        n296 = Add(x=w483, y=w484) -> (x+y=w482:i16)
        n297 = call <vilib>:"NT Write Number.vi"("Numeric"=w482, "Name"=w481) -> ()  [unwired: 9 in, 1 out]
      }
      event "Test Ring": Value Change {
        # "When a test mode helper value is selected from the ring,\nset the tree item's variable to the string value"
        n298 = event-data() -> ("NewVal"=w492:u16)  [unwired: 1 in]
        n299 = property on="Test Ring" class="Ring (strict)"() -> ("Strings []"=w493:string[])  [unwired: 2 in, 2 out]
        n300 = Index Array(array=w493, index=w492) -> (element=w491:string)
        n301 = call <vilib>:"NT Write String.vi"("String"=w491, "Name"=w490) -> ()  [unwired: 9 in, 1 out]
      }
      event "Rec Mode": Value Change {
        # "Update globals for recording mode and path to read log from.\nClear when logging and let NetworkTables set path for vision to\nuse."
        n302 = event-data() -> ("NewVal"=w505:enum32{"Stop", "Record", "Playback"})  [unwired: 1 in]
        n303 = global write "WPI_DashboardLogging Global.vi" "Logging Filename"(path "") -> ()
        n304 = global write "WPI_DashboardLogging Global.vi" "Recording"(w505) -> ()
        n305 = case shown="\"Playback\"" w505 {
          tunnel: w504 -> [_ w507 w516]
          tunnel: [_ _ w515] -> w501
          tunnel: [_ _ w514] -> _
          tunnel: w499 -> [_ _ w512]
          tunnel: cluster{i32, i32} {-250, 170} -> [_ _ w511]
          tunnel: [_ _ T25 {"Image Size"=TRUE, "Image Type"=TRUE, "Pixel Value"=TRUE, "ROI Information"=TRUE, "Zoom Factor"=FALSE} ("Image Information Shown:All Elements")] -> w497
          tunnel: [_ _ TRUE ("Zoom Factor")] -> w496
          tunnel: w495 -> [_ _ w508]
          frame Default {
          }
          frame "Stop", "Record" {
            # "Place Window too"
            n306 = invoke class="VI" method="FP.Close"(reference=w507) -> (reference out=w506:refnum<vi>)  [unwired: 2 in, 2 out]
            n307 = invoke class="VI" method="Abort VI"(reference=w506) -> ()  [unwired: 2 in, 3 out]
          }
          frame "Playback" {
            n308 = call "Open Playback Panel.vi"("Offset"=w511, "DB VI Ref"=w512, "Playback in"=w516) -> ("Playback out"=w513:refnum<vi>)  [unwired: 8 in]
            n309 = register-events(w513, w508) -> (reference out=w515:refnum<event-registration>, error out=w514:errorcluster)  [unwired: 2 in]
          }
        }
        n310 = property on="Camera Image" class="ImageControl"("Image Information Shown"=w497, "Image Information Visible"=w496) -> ()  [unwired: 2 in, 2 out]
        n311 = call <vilib>:"WPI_DashboardNT Log FieldName Cache.vi"("Operation"=enum16{"Lookup/Add", "Index", "Clear"}."Clear") -> ()  [unwired: 8 in, 3 out]
      }
      event Panel Close {
        w518 = enum32{"Stop", "Record", "Playback"}."Stop" ("Rec Mode")
        # "Playback window has been closed, abort"
        n312 = event-data() -> ()  [unwired: 1 in, 4 out]
        n313 = local write "Rec Mode"(w518) -> ()
        n314 = global write "WPI_DashboardLogging Global.vi" "Recording"(w518) -> ()
      }
      event Panel Close {
        # "Abort playback window and ourself"
        n315 = event-data() -> ()  [unwired: 1 in, 4 out]
        n316 = invoke class="VI" method="FP.Close"(reference=w524) -> (reference out=w523:refnum<vi>)  [unwired: 2 in, 2 out]
        n317 = invoke class="VI" method="Abort VI"(reference=w523) -> (error out=w522:errorcluster)  [unwired: 2 in, 2 out]
        n318 = invoke class="VI" method="Abort VI"(error in=w522) -> ()  [unwired: 2 in, 3 out]
      }
      event User Event {
        n319 = event-data() -> ("IDs"=w532:cluster{"RPC field ID":u16, "Unique ID":u16}, "String"=w531:string)  [unwired: 1 in]
        n320 = Bundle("IDs"=w532, "String"=w531) -> (w530:T11)  [unwired: 1 in]
        n321 = call <vilib>:"Retrieve RPC Response.vi"("RPC Response"=w530) -> ("Output"=w527:string[][])  [unwired: 10 in]
        n322 = Build Array (concatenate)(w525, w527) -> (w526:string[][])
        n323 = local write "Command Params"(w526) -> ()
        n324 = local write "Cmd Status"("" ("Cmd Status")) -> ()
      }
      event "Vision": Value Change {
        # "Enable/Disable Compression slider.\nHW USB is hard-coded into the camera"
        n325 = event-data() -> ("NewVal"=w539:u16)  [unwired: 1 in]
        n326 = Equal?(x=w539, y=u32 2 ("milliseconds to wait")) -> (x = y?=w537:bool)
        n327 = Select(t=T26."Disabled and Grayed Out" ("Disabled"), s=w537, f=T26."Enabled" ("Disabled")) -> (s? t:f=w534:T26)
        n328 = property on="Compression" class="Slide (strict)"("DisabledEnum"=w534) -> ()  [unwired: 2 in, 2 out]
      }
      event "Tree": Double Click {
        n329 = event-data() -> ("PlatMods"=w544:T29, "Tag"=w543:string)  [unwired: 1 in]
        n330 = Unbundle(w544) -> ("Shift"=w542:bool)  [unwired: 4 out]
        n331 = Not(x=w542) -> (.not. x?=w541:bool)
        n332 = call <vilib>:"NT Update Persistence.vi"("Persistence"=w541, "Name"=w543) -> ()  [unwired: 9 in, 1 out]
      }
    }
  }
  n333 = while {
    tunnel: w47 -> [w548]
    i -> [w551]
    stop <- FALSE stop-if-true
    n334 = Wait (ms)(milliseconds to wait=u32 100) -> ()  [unwired: 1 out]
    n335 = case shown="\"Playback\"" "Rec Mode" {
      tunnel: w551 -> [_ _ w566]
      tunnel: [u32 2829099 ("Base Color") u32 11141120 ("Target Color") w555] -> w547
      frame "Stop", Default {
        # "Reset the color, extra updates don't cost much"
      }
      frame "Record" {
      }
      frame "Playback" {
        # "Playback"
        n336 = Quotient & Remainder(x=w566, y=u32 50 ("milliseconds to wait")) -> (x-y*floor(x/y)=w562:u32)  [unwired: 1 out]
        n337 = Divide(x=w562, y=u32 50 ("milliseconds to wait")) -> (x/y=w559:dbl)
        n338 = Multiply(x=6.283185307179586, y=w559) -> (x*y=w564:dbl)
        n339 = Sine(x=w564) -> (sin(x)=w563:dbl)
        n340 = Absolute Value(x=w563) -> (abs(x)=w556:dbl)
        n341 = call "Interpolate RGB Color.vi"("Proportion"=w556, "Target Color"=u32 30976, "Base Color"=u32 2829099) -> ("Result Color"=w555:u32)  [unwired: 8 in]
      }
    }
    n342 = property class="Pane"(reference=w548, "PaneColor"=w547) -> ()  [unwired: 1 in, 2 out]
  }
  n343 = local write "Dashboard Tab"(T1."Drive" ("Dashboard Tab")) -> ()
  n344 = property on="On/Off" class="Bool (strict)"("Visible"=w15) -> ()  [unwired: 2 in, 2 out]
  n345 = property on="Motor" class="Clust (strict)"("Visible"=w15) -> ()  [unwired: 2 in, 2 out]
  n346 = property on="Progress" class="Clust (strict)"("Visible"=w15) -> ()  [unwired: 2 in, 2 out]
  n347 = property on="Test Ring" class="Ring (strict)"("Visible"=w15) -> ()  [unwired: 2 in, 2 out]
  n348 = property on="Rev/Fwd" class="Clust (strict)"("Visible"=w15) -> ()  [unwired: 2 in, 2 out]
  n349 = property on="Camera Settings" class="Clust (strict)"("Visible"=w15) -> ()  [unwired: 2 in, 2 out]
  n350 = while {
    tunnel: u16 1741 ("timeout ms (25000)") -> [w568]
    stop <- FALSE stop-if-true
    n351 = TCP Create Listener(10:w568) -> (0:w567:errorcluster, 3:w569:refnum<k5>)  [unwired: 4 in, 1 out]
    n352 = case shown="No Error" w567 {
      selector: w567 -> [w571 _]
      tunnel: w569 -> [w572 _]
      frame No Error {
        n353 = while {
          tunnel: w572 -> [w575]
          tunnel: w571 -> [w574]
          stop <- FALSE stop-if-true
          n354 = TCP Wait On Listener(8:w574, 11:w575) -> (0:w576:errorcluster, 4:w577:refnum<k5>)  [unwired: 2 in, 3 out]
          n355 = local write "TCP"(w577) -> ()
          n356 = case shown="No Error" w576 {
            frame No Error {
            }
            frame Error {
              n357 = Wait (ms)(milliseconds to wait=u32 1000) -> ()  [unwired: 1 out]
            }
          }
        }
      }
      frame Error {
        n358 = Wait (ms)(milliseconds to wait=u32 1000) -> ()  [unwired: 1 out]
      }
    }
  }
  n359 = local write "DB Camera Config"(w15) -> ()
  n360 = local write "Command Params"(string[][] [] ("Command Params")) -> ()
  n361 = global write "WPI_DashboardLogging Global.vi" "Recording"(w41) -> ()
  n362 = local write "Command Selection"(u16 0 ("milliseconds to wait")) -> ()
  n363 = local write "Rec Mode"(w41) -> ()
